vi "process.vi"(8 "error in (no error)":errorcluster, 9 "Calling VI Reference i":refnum<vi>, 10 "Node Refnum":refnum<vi>, 11 "Loop in":refnum<class "Loop.lvclass">) -> (0 "error out":errorcluster, 3 "Loop out":refnum<class "Loop.lvclass">)   [LabVIEW 2016, in "Loop.lvclass"]
uses:
  Loop.lvclass
  C:/LSST_TS/SystemSW/ct_tools/Node/Node.lvclass
  Dependency/Dependency.lvclass
  DiagramObject/DiagramObject.lvclass
  Node/Node.lvclass/Node.ctl
  DiagramObject/DiagramObject.lvclass/DiagramObject.ctl
  Dependency/Dependency.lvclass/Dependency.ctl
  Node/Node.lvclass
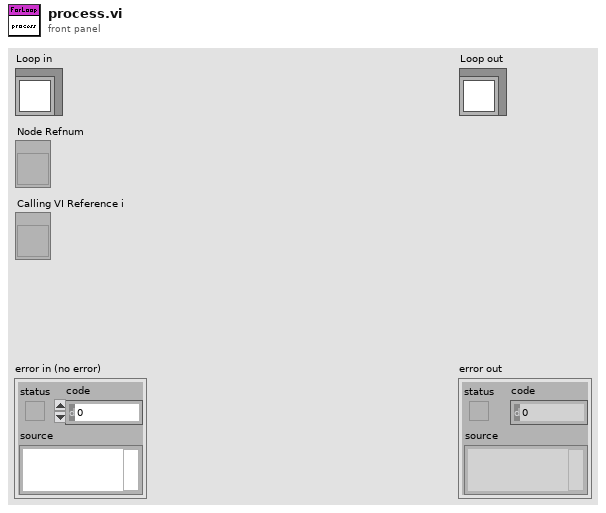
[diagram p1: front panel]
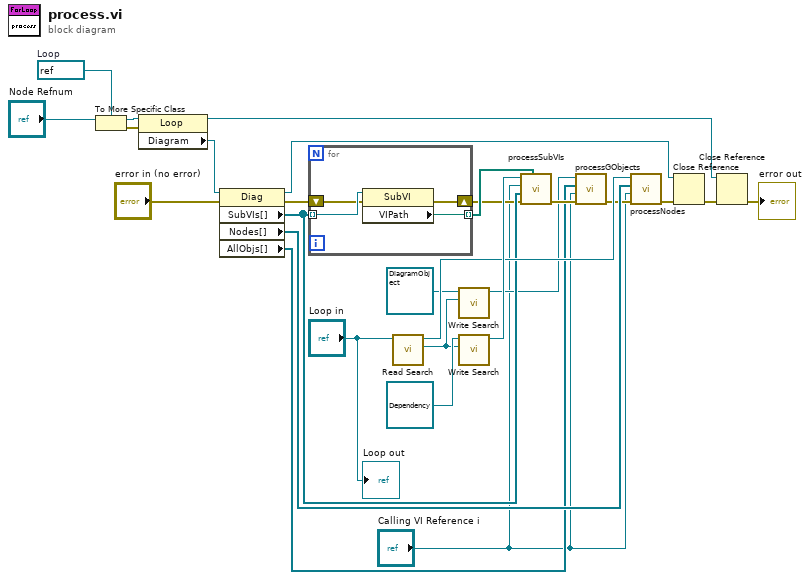
[diagram p0: block diagram]
diagram:
  w24 = refnum<vi> refnum  # Loop
  n1 = To More Specific Class(target class=w24, reference="Node Refnum") -> (specific class reference=w27:refnum<vi>, error out=w26:errorcluster)  [unwired: 1 in]
  n2 = property class="Loop"(reference=w27, error in=w26) -> (reference out=w22:refnum<vi>, "Diagram"=w25:refnum<vi>)  [unwired: 1 out]
  n3 = property class="Diag"(reference=w25, error in="error in (no error)") -> (reference out=w14:refnum<vi>, error out=w9:errorcluster, "SubVIs[]"=w11:refnum<vi>[], "Nodes[]"=w13:refnum<vi>[], "AllObjs[]"=w3:refnum<vi>[])
  n4 = for {
    tunnel: w11 -> [w31] mode=indexing
    tunnel: [w30] -> w10 mode=indexing
    shift-right: [w29] -> w8
    shift-left: w9 -> [w28]
    n5 = property class="SubVI"(reference=w31, error in=w28) -> (error out=w29:errorcluster, "VIPath"=w30:path)  [unwired: 1 out]
  }
  n6 = call "Read Search.vi"("Node in"="Loop in") -> ("Search"=w7:refnum<class "Search.lvclass">, "Node out"=w19:refnum<class "Loop.lvclass">)  [unwired: 9 in]
  n7 = call "Write Search.vi"("Search"=w7, "DiagramObject in"=refnum<class "DiagramObject.lvclass"> refnum ("DiagramObject.lvclass")) -> ("DiagramObject out"=w2:refnum<class "DiagramObject.lvclass">)  [unwired: 9 in]
  n8 = call "Write Search.vi"("Search"=w7, "Dependency in"=refnum<class "Dependency.lvclass"> refnum ("Dependency.lvclass")) -> ("Dependency out"=w20:refnum<class "Dependency.lvclass">)  [unwired: 9 in]
  n9 = call "processSubVIs.vi"("VIDependencyPaths"=w10, "error in (no error)"=w8, "SubVIs[]"=w11, "Calling VI Reference i"="Calling VI Reference i", "Dependency in"=w20) -> ("error out"=w5:errorcluster)  [unwired: 4 in, 2 out]
  n10 = call "processGObjects.vi"("error in (no error)"=w5, "Calling VI Reference i"="Calling VI Reference i", "All Objects[]"=w3, "DiagramObject in"=w2) -> ("error out"=w4:errorcluster)  [unwired: 6 in, 1 out]
  n11 = call "processNodes.vi"("error in (no error)"=w4, "Calling VI Reference i"="Calling VI Reference i", "Nodes[]"=w13, "Node in"=w19) -> ("error out"=w12:errorcluster)  [unwired: 6 in, 1 out]
  n12 = Close Reference(reference=w14, error in (no error)=w12) -> (error out=w23:errorcluster)
  n13 = Close Reference(reference=w22, error in (no error)=w23) -> (error out=→"error out":errorcluster)
  "Loop out" <- "Loop in"
